vi "_PID.vi"(0 "SetPoint":dbl=0.05, 1 "Kp":dbl=20.0, 2 "Ti":dbl=0.8, 3 "Sampling Time dt (s)":dbl=0.05 min=0.001 step=0.01 format="%#.3p", 4 "nivel":dbl=0.8) -> (5 "PI":dbl)   [LabVIEW 2010]
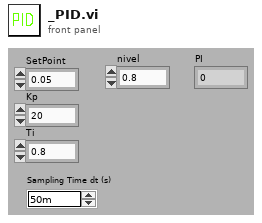
[diagram p1: front panel]
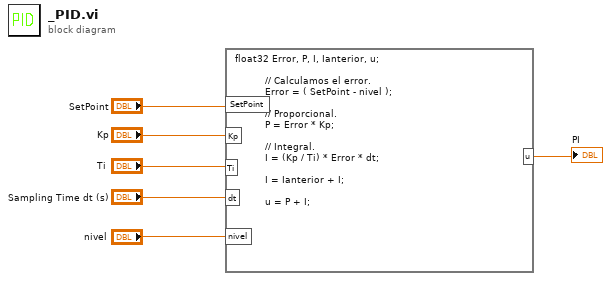
[diagram p0: block diagram]
diagram:
  n1 = formula code="float32 Error, P, I, Ianterior, u;\n          \n          // Calculamos el error.\n          Error = ( SetPoint - nivel );\n         \n          // Proporcional.\n          P = Error * Kp;    \n\n          // Integral. \n          I = (Kp / Ti) * Error * dt;\n\n          I = Ianterior + I;\n   \n          u = P + I;"("SetPoint"="SetPoint", "Kp"="Kp", "nivel"="nivel", "Ti"="Ti", "dt"="Sampling Time dt (s)") -> ("u"=→"PI":sgl)
